vi "plot -- LandauKhalat.vi"(7 "method":enum16{"max", "parab", "poly"}(ring), 9 "peaks":i32[](array[numeric]), 10 "cursor window out":T2={"left"=2044.0881763527054, "right "=2126.7657992565055, "center"=2085.4269878046052, "window"=82.67762290380006, "cursors"=[], "relative"=0, "absolute"=0, "fixed vertical offset"=2421.6740576496672, "vertical offset"=2421.6740576496672, "skew"=2421.6740576496672, "default window frac"=2421.6740576496672, "kind"=enum."fancy", "skew.left"=2.0, "skew.right"=0.0, "Plot ref"=refnum, "wing order"=enum."back"}, 11 "all unfiltered":T1(array[cluster])) -> (2 "Plot:   LandauKhalat":cluster{"Array":dbl[], dbl[]}[](graph))   [LabVIEW 2014]
uses:
  cursor winow.ctl
  <vilib>/Analysis/6fits.llb/Curve Fitting Criteria.ctl
  bylinear interpolation iiii- complex -- build matrix.vi
  <vilib>/Analysis/baseanly.llb/A x B.vi
  <vilib>/Analysis/baseanly.llb/Complex A x B.vi
  parabola -- complex.vi
  Q -- check range -- i -- real.vi
  line -- complex.vi
  Q -- check range -- i -- integer.vi
  Q - not nan -- real.vi
  Q - not nan -- integer.vi
  <vilib>/Analysis/Matrix/Numeric/Conversions/Array To Matrix.vi
  <vilib>/Analysis/Matrix/Numeric/Conversions/Array To Matrix - RA2.vi
  <vilib>/Analysis/baseanly.llb/Inverse Matrix.vi
  <vilib>/Analysis/baseanly.llb/Real Inverse Matrix.vi
  <vilib>/Analysis/NI_AALPro.lvlib
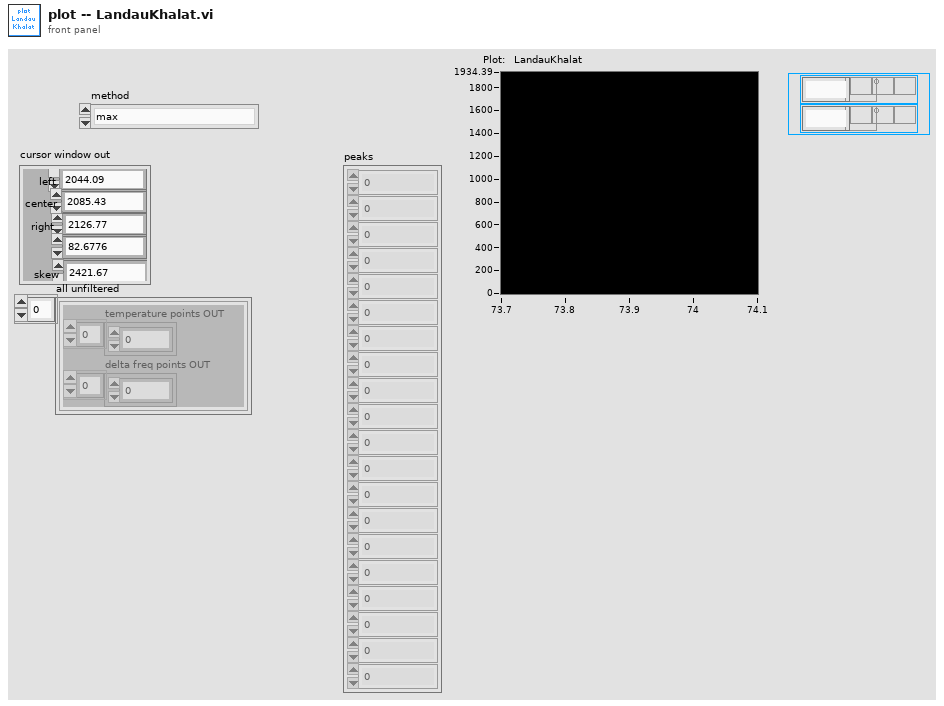
[diagram p1: front panel]
types:
  T1 = cluster{"temperature points OUT":dbl[], "delta freq points OUT":dbl[]}[]
  T2 = typedef "cursor winow.ctl" = cluster{"left":dbl, "right ":dbl, "center":dbl, "window":dbl, "cursors":i32[], "relative":i32, "absolute":i32, "fixed vertical offset":dbl, "vertical offset":dbl, "skew":dbl, "default window frac":dbl, "kind":enum16{"symmetric", "skewed", "fancy"}, "skew.left":dbl, "skew.right":dbl, "Plot ref":refnum<vi>, "wing order":enum16{"forw", "back"}}
  T3 = typedef "NI_AALPro.lvlib/Curve Fitting Criteria.ctl" = u16
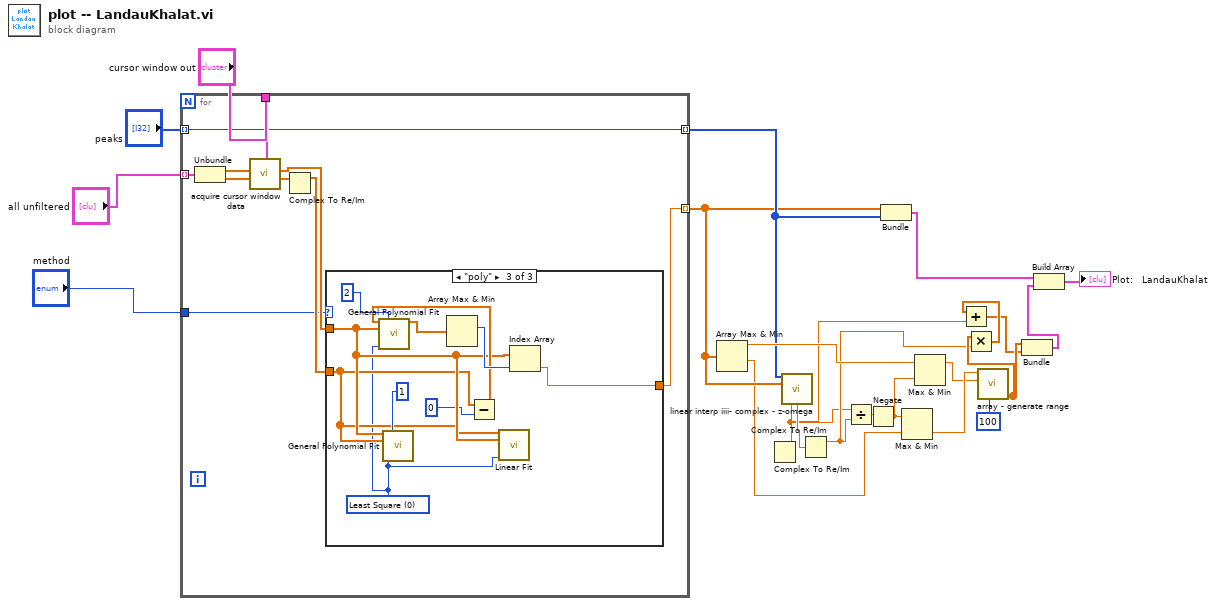
[diagram p0: block diagram]
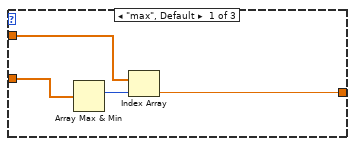
[diagram p2: hidden frame]
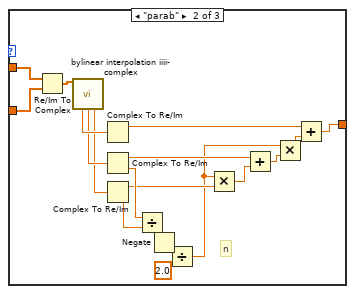
[diagram p3: hidden frame]
diagram:
  n1 = for {
    tunnel: "all unfiltered" -> [w33] mode=indexing
    tunnel: "peaks" -> [w28] mode=indexing
    tunnel: "cursor window out" -> [w32]
    tunnel: [w25] -> w14 mode=indexing
    tunnel: [w28] -> w15 mode=indexing
    tunnel: "method" -> [w24]
    n2 = Unbundle(w33) -> ("temperature points OUT"=w31:dbl[], "delta freq points OUT"=w30:dbl[])
    n3 = call "acquire cursor window data.vi"("z in"=w30, "omega in"=w31, "cursor window"=w32) -> ("z out"=w29:cdb[], "omega  out"=w27:dbl[])  [unwired: 4 in, 3 out]
    n4 = Complex To Re/Im(x + iy=w29) -> (x=w26:dbl[])  [unwired: 1 out]
    n5 = case shown="\"poly\"" w24 {
      tunnel: w27 -> [w36 w56 w60]
      tunnel: w26 -> [w35 w55 w59]
      tunnel: [w34 w38 w63] -> w25
      frame "max", Default {
        n6 = Array Max & Min(array=w35) -> (max index (indices)=w37:i32)  [unwired: 3 out]
        n7 = Index Array(array=w36, index=w37) -> (element=w34:dbl)
      }
      frame "parab" {
        # "n"
        n8 = Re/Im To Complex(1:w55, 2:w56) -> (0:w54:cdb[])
        n9 = call "bylinear interpolation iiii- complex.vi"("Array"=w54) -> ("intercept"=w53:cdb, "slope"=w52:cdb, "curvature"=w51:cdb)  [unwired: 4 in, 8 out]
        n10 = Complex To Re/Im(x + iy=w53) -> (x=w39:dbl)  [unwired: 1 out]
        n11 = Complex To Re/Im(x + iy=w52) -> (x=w43:dbl, y=w49:dbl)
        n12 = Complex To Re/Im(x + iy=w51) -> (x=w45:dbl, y=w48:dbl)
        n13 = Divide(x=w49, y=w48) -> (x/y=w50:dbl)
        n14 = Negate(x=w50) -> (-x=w47:dbl)
        n15 = Divide(x=w47, y=2.0) -> (x/y=w41:dbl)
        n16 = Multiply(x=w41, y=w45) -> (x*y=w44:dbl)
        n17 = Add(x=w43, y=w44) -> (x+y=w42:dbl)
        n18 = Multiply(x=w41, y=w42) -> (x*y=w40:dbl)
        n19 = Add(x=w39, y=w40) -> (x+y=w38:dbl)
      }
      frame "poly" {
        w58 = T3 0 items=["Least Square", "Least Absolute Residual", "Bisquare"] ("method")
        n20 = call <vilib>:"General Polynomial Fit.vi"("Y"=w60, "polynomial order"=1, "X"=w59, "method"=w58) -> ()  [unwired: 8 in, 4 out]
        n21 = Subtract(x=w59, y=0 ("polynomial order")) -> (x-y=w61:dbl[])
        n22 = call <vilib>:"General Polynomial Fit.vi"("Y"=w61, "polynomial order"=2, "X"=w60, "method"=w58) -> ("Best Polynomial Fit"=w65:dbl[])  [unwired: 8 in, 3 out]
        n23 = Array Max & Min(array=w65) -> (max index (indices)=w64:i32)  [unwired: 3 out]
        n24 = call <vilib>:"Linear Fit.vi"("Y"=w59, "X"=w60, "method"=w58) -> ()  [unwired: 8 in, 5 out]
        n25 = Index Array(array=w60, index=w64) -> (element=w63:dbl)
      }
    }
  }
  n26 = Array Max & Min(array=w14) -> (max value=w20:dbl, min value=w1:dbl)  [unwired: 2 out]
  n27 = call "linear interp iiii- complex - z-omega.vi"("z"=w15, "omega"=w14) -> ("intercept"=w22:cdb, "slope"=w21:cdb)  [unwired: 5 in, 7 out]
  n28 = Complex To Re/Im(x + iy=w22) -> (x=w8:dbl)  [unwired: 1 out]
  n29 = Complex To Re/Im(x + iy=w21) -> (x=w10:dbl)  [unwired: 1 out]
  n30 = Divide(x=w8, y=w10) -> (x/y=w23:dbl)
  n31 = Negate(x=w23) -> (-x=w19:dbl)
  n32 = Bundle(w14, w15) -> (w12:cluster{dbl[], i32[]})  [unwired: 1 in]
  n33 = Max & Min(x=w19, y=w1) -> (min(x,y)=w18:dbl)  [unwired: 1 out]
  n34 = Max & Min(x=w20, y=w19) -> (max(x,y)=w17:dbl)  [unwired: 1 out]
  n35 = call "array - generate range.vi"("N"=100, "freq max"=w17, "freq min"=w18) -> ("Array"=w11:dbl[])  [unwired: 7 in, 1 out]
  n36 = Multiply(x=w11, y=w10) -> (x*y=w9:dbl[])
  n37 = Add(x=w9, y=w8) -> (x+y=w7:dbl[])
  n38 = Bundle("Array"=w11, w7) -> (w6:cluster{"Array":dbl[], dbl[]})  [unwired: 1 in]
  n39 = Build Array(w12, w6) -> (→"Plot:   LandauKhalat":cluster{"Array":dbl[], dbl[]}[])
